vi "Get Workflows.vi"(11 "Workflows In":string) -> (3 "Workflow Map":map{string, string[]}(c390))   [LabVIEW 2021]
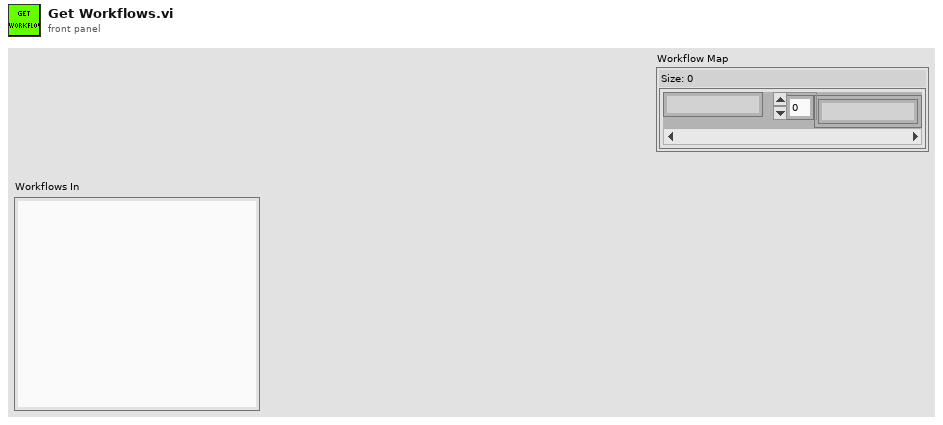
[diagram p1: front panel]
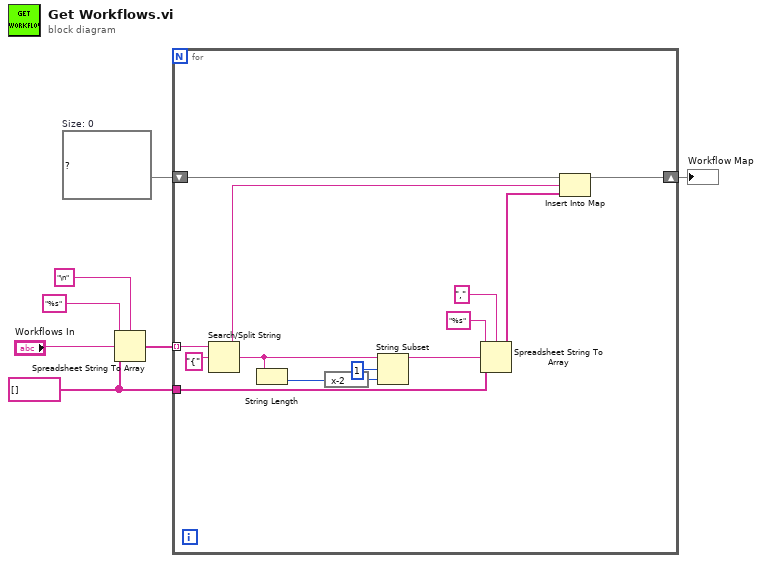
[diagram p0: block diagram]
diagram:
  w2 = map{string, string[]} {}  # Size: 0
  w3 = string[] []
  n1 = Spreadsheet String To Array(delimiter (Tab)="\n", format string="%s", spreadsheet string="Workflows In", array type (2D Dbl)=w3) -> (array=w4:string[])
  n2 = for {
    tunnel: w4 -> [w21] mode=indexing
    tunnel: w3 -> [w17]
    shift-right: [w10] -> w1
    shift-left: w2 -> [w11]
    n3 = Search/Split String(string=w21, search string/char (-)="{") -> (substring before match=w9:string, match + rest of string=w14:string)  [unwired: 1 in, 1 out]
    n4 = String Length(string=w14) -> (length=w13:i32)
    n5 = expression code="x-2"(w13) -> (w12:i32)
    n6 = String Subset(string=w14, offset (0)=1, length (rest)=w12) -> (substring=w16:string)
    n7 = Spreadsheet String To Array(delimiter (Tab)=",", format string="%s", spreadsheet string=w16, array type (2D Dbl)=w17) -> (array=w8:string[])
    n8 = Insert Into Map(map in=w11, key=w9, value=w8) -> (map out=w10:map{string, string[]})  [unwired: 2 out]
  }
  "Workflow Map" <- w1
